vi "JLINK DownloadFile.vi"(8 "error in (no error)":errorcluster, 10 "Prog. addr. (bin file only)":u32 format="0x%08x", 11 "File Path":string) -> (0 "error out":errorcluster, 3 "Return value":i32)   [LabVIEW 2020, in "JLinkARM.lvlib"]
uses:
  Lib/JLinkARM.lvlib
  JLinkARM.dll
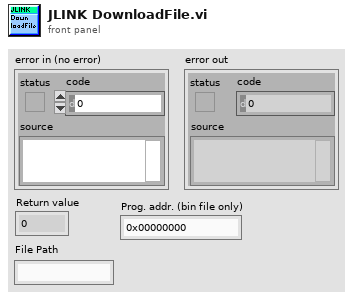
[diagram p1: front panel]
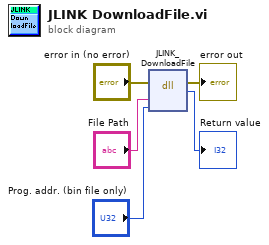
[diagram p0: block diagram]
diagram:
  n1 = dll-call lib="C:/Users/anybody/Desktop/JLinkARM.dll" fn="JLINK_DownloadFile"(error in="error in (no error)", "sFileName"="File Path", "Addr"="Prog. addr. (bin file only)") -> (error out=→"error out":errorcluster, "return type"=→"Return value":i32)  [unwired: 4 in, 1 out]
